vi "Feeder Controller.vi"(8 "error in":errorcluster) -> ()   [LabVIEW 2019]
doc: "This VI executes continuously carrying out the current operation and responding to updates or new operations. It will often contain the timing or control code that is difficult to place directly in TeleOp. This VI generally opens all sensors and motors and isolates the rest of the robot code from knowing how the operations are carried out."
uses:
  <vilib>/Rock Robotics/WPI/Framework/Completion Status.ctl
  Feeder Setpoints.ctl
  Feeder Operations.ctl
  <vilib>/Rock Robotics/WPI/ThirdParty/REV Robotics/SPARK MAX/Typedef/Spark MAX Control Type.ctl
  Feeder Published Globals.vi
  Framework/Robot Global Data.vi
  <vilib>/Rock Robotics/Network Tables/NT Write Boolean.vi
panel:
  out "Setpoints":T1(graph)
  out "Feeder Velocity":T2(graph)
  in  "Motor CAN IDs":cluster{"Feeder":u8, "Index":u8}={"Feeder"=11, "Index"=9}
  in  "Interactive Values":T3
  out "Current\nCmd":string
  in  "Buttons":cluster{"Execute Cmd":bool, "Abort Cmd":bool}
  out "Command Timing":cluster{"Start Time (ms)":u32, "Iterations":i32}
  out "Status":T5
  # "Click here to set min"
  # "Interactive Command: You may fill in the settings for a command\nand schedule it with the Execute button. You can observe and abort\nany command while fine tuning the code for the controller."
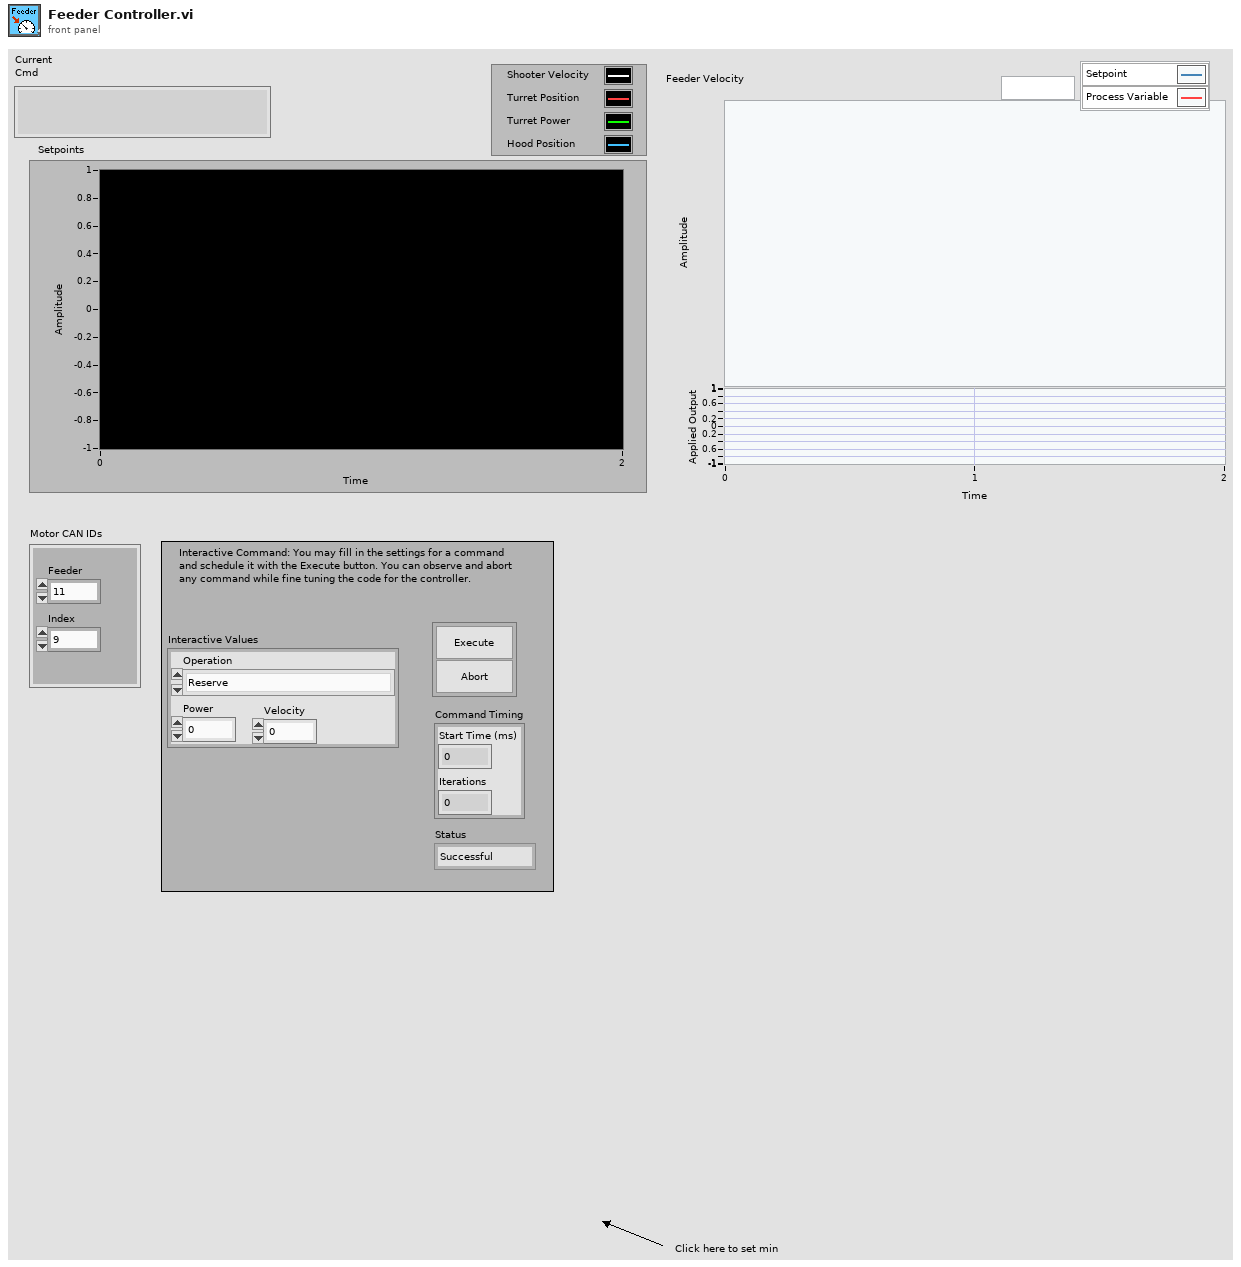
[diagram p1: front panel]
types:
  T1 = cluster{"Velocity Setpoint":dbl, "Power Setpoint":dbl, "output":dbl, "output 2":dbl}
  T2 = cluster{"Sensor Velocity":dbl, "Setpoint":dbl, "Applied Output":dbl}
  T3 = typedef "Feeder Setpoints.ctl" = cluster{"Operation":T4, "Power":dbl, "Velocity":dbl}
  T4 = typedef "Feeder Operations.ctl" = enum16{"Reserve", "Read Current", "Immediate", "Index Out Immediate", "Index In Immediate", "Start Feeder", "Stop Feeder"}
  T5 = typedef "Completion Status.ctl" = enum16{"Successful", "Aborted", "Incomplete"}
  T6 = typedef "WPI_MotorControlDeviceRef.ctl" = cluster{"DeviceStatus":errorcluster, "Type":T7, "PWM":cluster{"PWM Channel":T8, "DeadBand":T9}, "CAN":cluster{"Device Number":u8, "SetOutput VI Ref":variant, "GetOutput VI Ref":variant, "Enable VI Ref":variant, "Disable VI Ref":variant, "Data":variant}, "Invert":bool, "DIO PWM":cluster{"PWM \"Enable\" Channel":T8, "DIOChannel":T10, "PWM Rate":dbl}}
  T7 = typedef "WPI_MotorControlType.ctl" = enum16{"PWM", "CAN", "DIO PWM"}
  T8 = typedef "FPGA_DIOPWMChannel.ctl" = enum8{"PWM 0", "PWM 1", "PWM 2", "PWM 3", "PWM 4", "PWM 5", "PWM 6", "PWM 7", "PWM 8", "PWM 9", "PWM MXP 0", "PWM MXP 1", "PWM MXP 2", "PWM MXP 3", "PWM MXP 4", "PWM MXP 5", "PWM MXP 6", "PWM MXP 7", "PWM MXP 8", "PWM MXP 9", "Invalid"}
  T9 = typedef "WPI_PWMDeadband.ctl" = cluster{"Name":string, "maxPositivePwm":i32, "minPositivePwm":i32, "centerPwm":i32, "maxNegativePwm":i32, "minNegativePwm":i32, "angularRange":u16}
  T10 = typedef "FPGA_DIOChannel.ctl" = enum8{"DIO 0", "DIO 1", "DIO 2", "DIO 3", "DIO 4", "DIO 5", "DIO 6", "DIO 7", "DIO 8", "DIO 9", "DIO MXP 0", "DIO MXP 1", "DIO MXP 2", "DIO MXP 3", "DIO MXP 4", "DIO MXP 5", "DIO MXP 6", "DIO MXP 7", "DIO MXP 8", "DIO MXP 9", "DIO MXP 10", "DIO MXP 11", "DIO MXP 12", "DIO MXP 13", "DIO MXP 14", "DIO MXP 15", "SPI Port CS1", "SPI Port CS2", "SPI Port CS3", "SPI Port MISO", "SPI Port MOSI", "Invalid"}
  T11 = typedef "Command Status Info.ctl" = cluster{"Name":string, "Status":T5, "notifier out":T12}
  T12 = typedef "Completion Notifier.ctl" = refnum<notifier>
  T13 = cluster{"Current Command":T3, "Command Timing":cluster{"Start Time (ms)":u32, "Iterations":i32}, "Command Arguments":cluster{"Command Info":T11, "Description":string, "Default Command":T3, "queue out":refnum<queue>, "Subsystem Name":string}}
  T14 = typedef "Spark MAX Control Type.ctl" = enum16{"Percent VBus", "Voltage", "Velocity", "Position", "Smart Motion", "Current", "Smart Velocity"}
  T15 = cluster{"P Gain":dbl, "I Gain":dbl, "D Gain":dbl, "F Gain":dbl, "I Zone":dbl, "Min Output":dbl, "Max Output":dbl}
  T16 = cluster{dbl, "Velocity":dbl, "Applied Output":dbl}
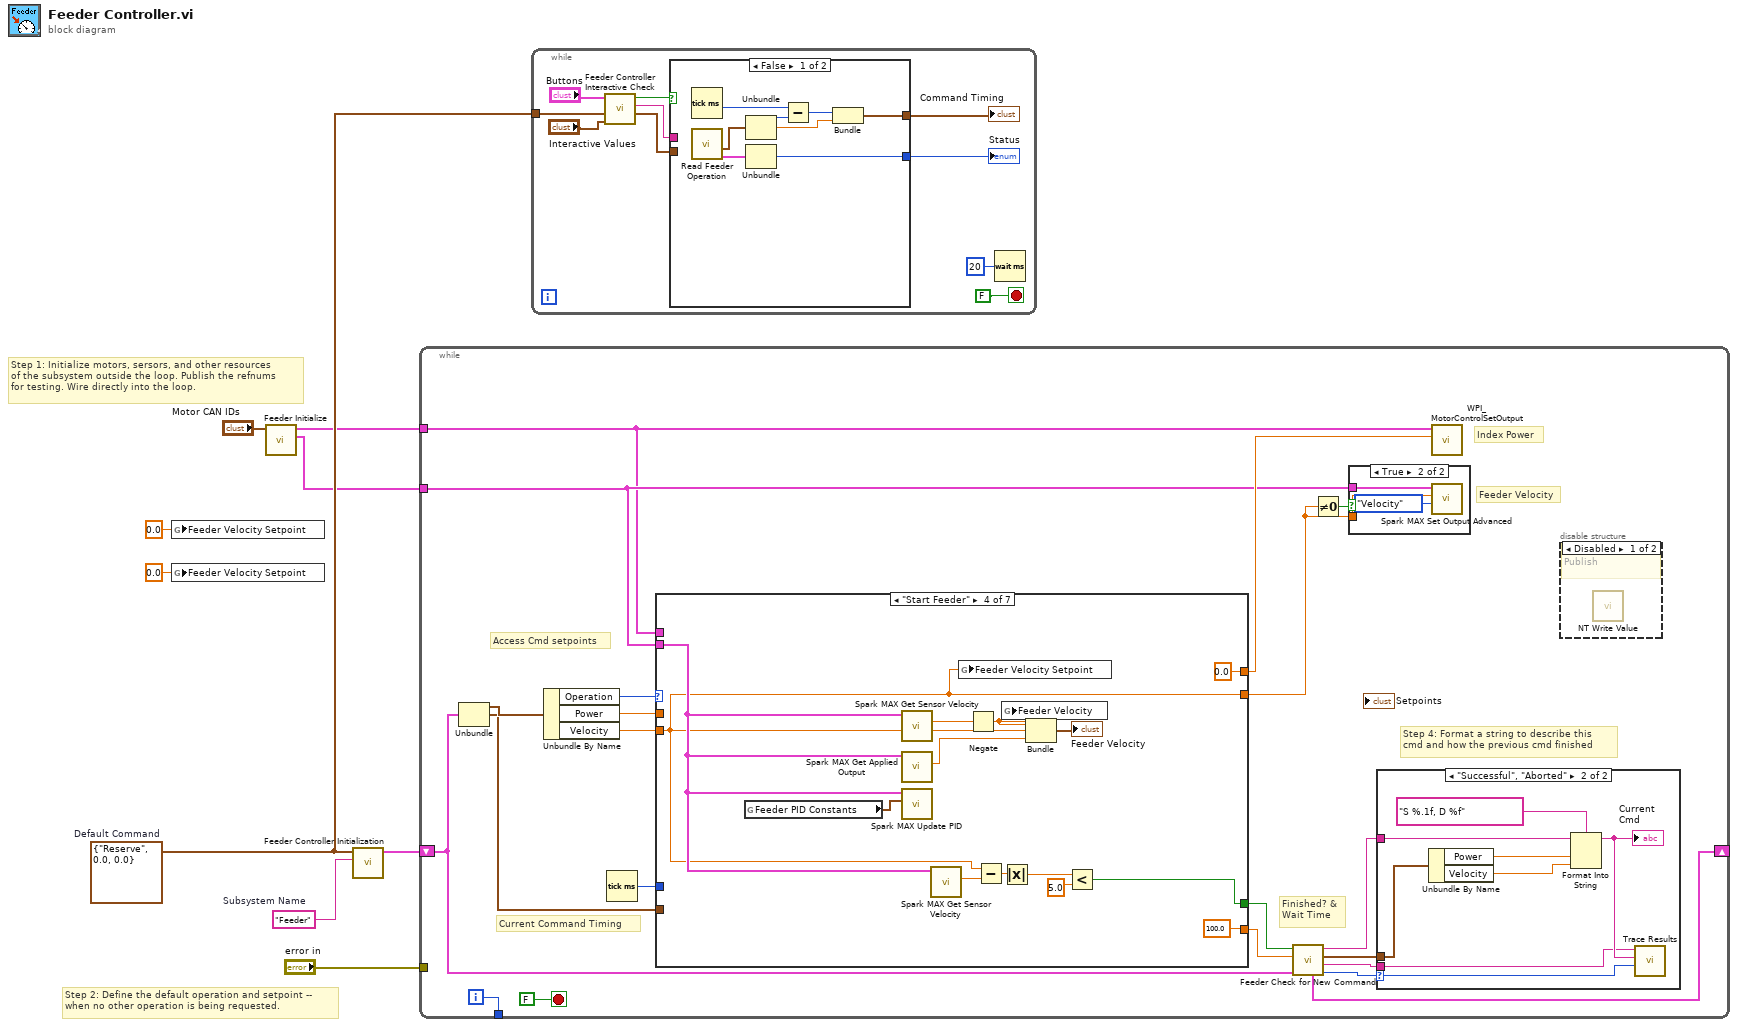
[diagram p0: block diagram]
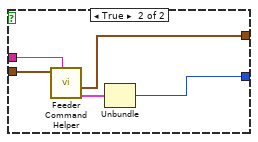
[diagram p2: hidden frame]
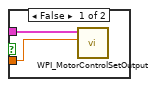
[diagram p3: hidden frame]
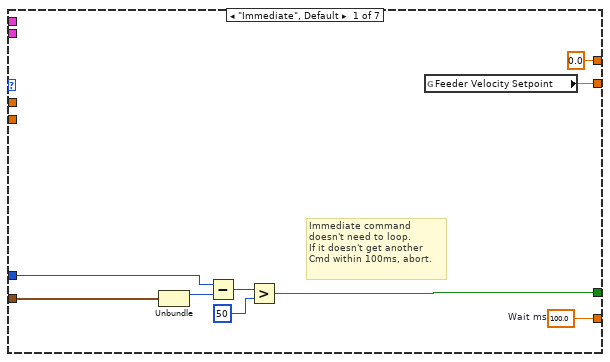
[diagram p6: hidden frame]
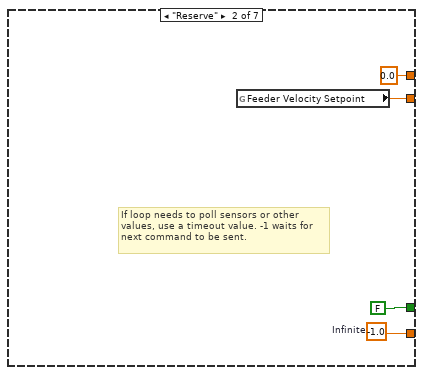
[diagram p7: hidden frame]
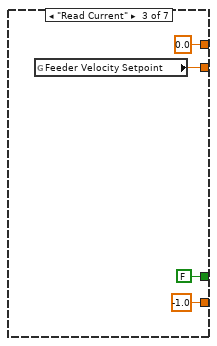
[diagram p8: hidden frame]
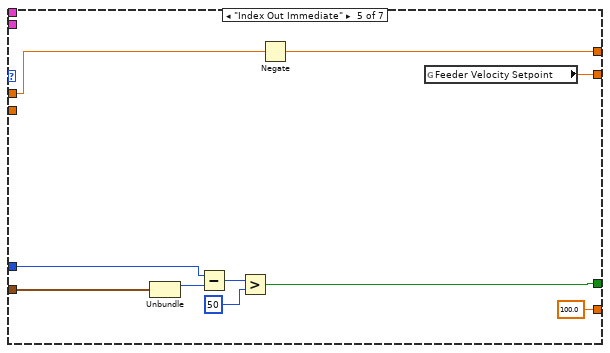
[diagram p9: hidden frame]
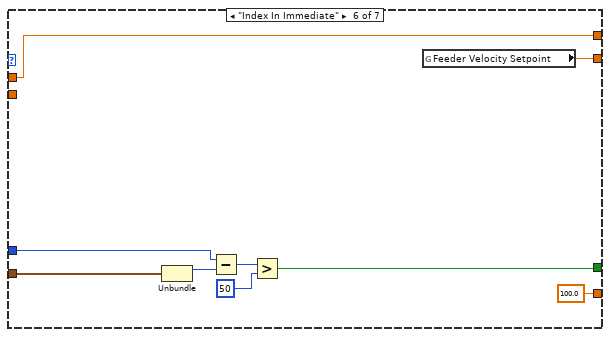
[diagram p10: hidden frame]
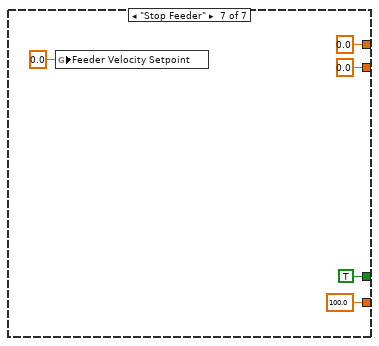
[diagram p11: hidden frame]
diagram:
  w6 = T3 {"Operation"=enum."Reserve", "Power"=0.0, "Velocity"=0.0}  # Default Command
  w7 = "Feeder"  # Subsystem Name
  # "Step 2: Define the default operation and setpoint --\nwhen no other operation is being requested."
  # "Step 1: Initialize motors, sersors, and other resources\nof the subsystem outside the loop. Publish the refnums\nfor testing. Wire directly into the loop."
  n1 = global write "Feeder Published Globals.vi" "Feeder Velocity Setpoint"(0.0 ("Feeder Velocity Setpoint")) -> ()
  n2 = global write "Feeder Published Globals.vi" "Feeder Velocity Setpoint"(0.0 ("Feeder Velocity Setpoint")) -> ()
  n3 = call "Feeder Initialize.vi"("Motor CAN IDs"="Motor CAN IDs") -> ("MotorControlDeviceRef"=w3:T6, "MotorControlDeviceRef 2"=w5:T6)  [unwired: 9 in]
  n4 = call "Feeder Controller Initialization.vi"("Subsystem Name"=w7, "Default Command"=w6) -> ("Current Command"=w8:T13)  [unwired: 9 in]
  n5 = while {
    shift-right: [w24] -> _
    shift-left: w8 -> [w17]
    tunnel: [w29] -> _
    tunnel: "error in" -> [_]
    tunnel: w5 -> [w12]
    tunnel: w3 -> [w13]
    i -> [w29]
    stop <- FALSE stop-if-true
    # "Feeder Velocity"
    # "Index Power"
    # "Step 4: Format a string to describe this\ncmd and how the previous cmd finished"
    # "Current Command Timing"
    # "Access Cmd setpoints"
    # "Finished? &\nWait Time"
    n6 = Unbundle(w17) -> ("Current Command"=w28:T3, "Command Timing"=w26:cluster{"Start Time (ms)":u32, "Iterations":i32})  [unwired: 1 out]
    n7 = Unbundle By Name(w28) -> ("Operation"=w14:T4, "Power"=w25:dbl, "Velocity"=w15:dbl)
    n8 = Tick Count (ms)() -> (millisecond timer value=w27:u32)
    n9 = case shown="\"Start Feeder\"" w14 {
      tunnel: [w52 w56 -1.0 ("Infinite") 100.0 ("Infinite") 100.0 ("Infinite") 100.0 ("Infinite") 100.0 ("Infinite")] -> w22
      tunnel: [w46 FALSE ("ignore previous (F)") FALSE ("ignore previous (F)") w64 w78 w89 TRUE ("ignore previous (F)")] -> w23
      tunnel: w26 -> [w48 _ _ _ w79 w90 _]
      tunnel: w27 -> [w47 _ _ _ w76 w86 _]
      tunnel: w25 -> [_ _ _ _ w84 w87 _]
      tunnel: [0.0 ("Power") 0.0 ("Power") 0.0 ("Power") 0.0 ("Power") w83 w87 0.0 ("Power")] -> w16
      tunnel: w15 -> [_ _ _ w63 _ _ _]
      tunnel: w12 -> [_ _ _ _ _ _ _]
      tunnel: w13 -> [_ _ _ w65 _ _ _]
      tunnel: [w45 w54 w59 w63 w75 w85 0.0 ("Velocity")] -> w10
      frame "Immediate", Default {
        w52 = 100.0  # Wait ms
        # "Immediate command\ndoesn't need to loop.\nIf it doesn't get another\nCmd within 100ms, abort."
        n10 = Unbundle(w48) -> ("Start Time (ms)"=w51:u32)  [unwired: 1 out]
        n11 = Subtract(x=w47, y=w51) -> (x-y=w50:u32)
        n12 = Greater?(x=w50, y=u8 50 ("Left Motor")) -> (0:w46:bool)
        n13 = global read "Feeder Published Globals.vi" "Feeder Velocity Setpoint"() -> (w45:dbl)
      }
      frame "Reserve" {
        w56 = -1.0  # Infinite
        # "If loop needs to poll sensors or other\nvalues, use a timeout value. -1 waits for\nnext command to be sent."
        n14 = global read "Feeder Published Globals.vi" "Feeder Velocity Setpoint"() -> (w54:dbl)
      }
      frame "Read Current" {
        n15 = global read "Feeder Published Globals.vi" "Feeder Velocity Setpoint"() -> (w59:dbl)
      }
      frame "Start Feeder" {
        n16 = global read "Feeder Published Globals.vi" "Feeder PID Constants"() -> (w72:T15)
        n17 = call <vilib>:"Spark MAX Get Sensor Velocity.vi"("MotorControlDevRef in"=w65) -> ("Sensor Velocity"=w62:dbl)  [unwired: 7 in, 3 out]
        n18 = call <vilib>:"Spark MAX Get Applied Output.vi"("MotorControlDevRef in"=w65) -> ("Applied Output"=w71:dbl)  [unwired: 7 in, 3 out]
        n19 = call "Spark MAX Update PID.vi"("MotorControlDeviceRef"=w65, "PID Constants"=w72) -> ()  [unwired: 8 in]
        n20 = call <vilib>:"Spark MAX Get Sensor Velocity.vi"("MotorControlDevRef in"=w65) -> ("Sensor Velocity"=w68:dbl)  [unwired: 7 in, 3 out]
        n21 = global write "Feeder Published Globals.vi" "Feeder Velocity Setpoint"(w63) -> ()
        n22 = Negate(x=w62) -> (-x=w61:dbl)
        n23 = Subtract(x=w63, y=w68) -> (x-y=w69:dbl)
        n24 = global write "Robot Global Data.vi" "Feeder Velocity"(w61) -> ()
        n25 = Absolute Value(x=w69) -> (abs(x)=w67:dbl)
        n26 = Bundle(w61, "Velocity"=w63, "Applied Output"=w71) -> (→"Feeder Velocity":T16)  [unwired: 1 in]
        n27 = Less?(x=w67, y=5.0) -> (x < y?=w64:bool)
      }
      frame "Index Out Immediate" {
        n28 = Unbundle(w79) -> ("Start Time (ms)"=w81:u32)  [unwired: 1 out]
        n29 = Subtract(x=w76, y=w81) -> (x-y=w82:u32)
        n30 = Greater?(x=w82, y=u8 50 ("Left Motor")) -> (0:w78:bool)
        n31 = Negate(x=w84) -> (-x=w83:dbl)
        n32 = global read "Feeder Published Globals.vi" "Feeder Velocity Setpoint"() -> (w75:dbl)
      }
      frame "Index In Immediate" {
        n33 = Unbundle(w90) -> ("Start Time (ms)"=w93:u32)  [unwired: 1 out]
        n34 = Subtract(x=w86, y=w93) -> (x-y=w92:u32)
        n35 = Greater?(x=w92, y=u8 50 ("Left Motor")) -> (0:w89:bool)
        n36 = global read "Feeder Published Globals.vi" "Feeder Velocity Setpoint"() -> (w85:dbl)
      }
      frame "Stop Feeder" {
        n37 = global write "Feeder Published Globals.vi" "Feeder Velocity Setpoint"(0.0 ("Feeder Velocity Setpoint")) -> ()
      }
    }
    n38 = call "Feeder Check for New Command.vi"("Current Command"=w17, "Wait time (ms)"=w22, "Finished?"=w23) -> ("Completion"=w18:T5, "Subsystem Name"=w19:string, "Current Command"=w20:T3, "Initial Trace String"=w21:string, "NextCommand"=w24:T13)  [unwired: 4 in]
    n39 = Not Equal To 0?(x=w10) -> (x != 0?=w11:bool)
    n40 = case shown="True" w11 {
      tunnel: w13 -> [w32 w35]
      tunnel: w10 -> [w31 w34]
      frame False {
        n41 = call <vilib>:"WPI_MotorControlSetOutput.vi"("Output"=w31, "MotorControlDevRef"=w32) -> ()  [unwired: 7 in, 3 out]
      }
      frame True {
        n42 = call <vilib>:"Spark MAX Set Output Advanced.vi"("Control Mode"=Spark_MAX_Control_Type."Velocity", "Setpoint"=w34, "MotorControlDevRef"=w35) -> ()  [unwired: 7 in, 2 out]
      }
    }
    n43 = case shown="\"Successful\", \"Aborted\"" w18 {
      selector: w18 -> [_ w43]
      tunnel: w21 -> [_ w39]
      tunnel: w20 -> [_ w40]
      tunnel: w19 -> [_ w36]
      frame "Incomplete", Default {
        # "Continuing current command"
      }
      frame "Successful", "Aborted" {
        # "Report and setup for next command"
        n44 = Unbundle By Name(w40) -> ("Power"=w42:dbl, "Velocity"=w37:dbl)
        n45 = Format Into String(format string="S %.1f, D %f", initial string=w39, w42, w37) -> (resulting string=w38:string)  [unwired: 1 in, 1 out]
        "Current\nCmd" <- w38
        n46 = call <vilib>:"Trace Results.vi"("Status of previous command"=w43, "Description"=w38, "Subsystem"=w36) -> ()  [unwired: 9 in]
      }
    }
    n47 = call <vilib>:"WPI_MotorControlSetOutput.vi"("Output"=w16, "MotorControlDevRef"=w12) -> ()  [unwired: 7 in, 3 out]
    n48 = disable-structure shown="Disabled" {
      frame Disabled {
        # "Publish"
        n49 = call-poly <vilib>:"NT Write Value.vi"() -> ()  [unwired: 11 in, 1 out]
      }
      frame Enabled {
      }
    }
  }
  n50 = while {
    tunnel: w6 -> [w105]
    stop <- FALSE stop-if-true
    n51 = call "Feeder Controller Interactive Check.vi"("Interactive Command in"="Interactive Values", "Default Command"=w105, "Buttons"="Buttons") -> ("Interactive Command out"=w102:T3, "Trace String"=w103:string, "Schedule"=w104:bool)  [unwired: 6 in]
    n52 = case shown="False" w104 {
      tunnel: [w116 w121] -> w101
      tunnel: w102 -> [_ w119]
      tunnel: [w112 w117] -> w100
      tunnel: w103 -> [_ w120]
      frame False {
        n53 = Tick Count (ms)() -> (millisecond timer value=w111:u32)
        n54 = call "Read Feeder Operation.vi"() -> ("Command Info"=w109:T11, "SubSystem Data"=w110:T3)  [unwired: 9 in, 1 out]
        n55 = Unbundle(w110) -> ("Operation"=w115:T4, "Power"=w113:dbl)  [unwired: 1 out]
        n56 = Unbundle(w109) -> ("Status"=w116:T5)  [unwired: 2 out]
        n57 = Subtract(x=w111, y=w115) -> (x-y=w114:u32)
        n58 = Bundle(w114, "Power"=w113) -> (w112:cluster{u32, "Power":dbl})  [unwired: 1 in]
      }
      frame True {
        n59 = call "Feeder Command Helper.vi"("Description"=w120, "SubSystem Data"=w119) -> ("Command Info Out"=w118:T11, "Command Timing"=w117:cluster{"Start Time (ms)":u32, "Iterations":i32})  [unwired: 7 in, 1 out]
        n60 = Unbundle(w118) -> ("Status"=w121:T5)  [unwired: 2 out]
      }
    }
    "Status" <- w101
    "Command Timing" <- w100
    n61 = Wait (ms)(milliseconds to wait=u32 20) -> ()  [unwired: 1 out]
  }
